vi "Start Battle.vi"(11 "Board Size":i32) -> (0 "Start":bool=TRUE)   [LabVIEW 2015, in "SB SubVIs.lvlib"]
uses:
  SB SubVIs.lvlib
  Type Defs/Square Cluster.ctl
  Square/Square.lvclass
  Globals.vi
  Globals (private).vi
  Type Defs/SB Type Defs.lvlib
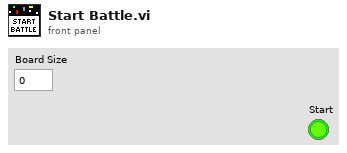
[diagram p1: front panel]
types:
  T1 = typedef "SB Type Defs.lvlib/Square Cluster.ctl" = cluster{"Attacked":bool, "Team":i32, "Next Turn":i32, "DVR":refnum<data-value>}
  T2 = typedef "SB Type Defs.lvlib/UI Refs.ctl" = cluster{"Battlefield":refnum<vi>, "Dashboard":refnum<vi>, "End Battle":refnum<vi>, "Time Limit":refnum<vi>}
  T3 = typedef "SB Type Defs.lvlib/Dashboard.ctl" = cluster{"Color":u32, "Player":i32, "Status":string, "Stats":string}
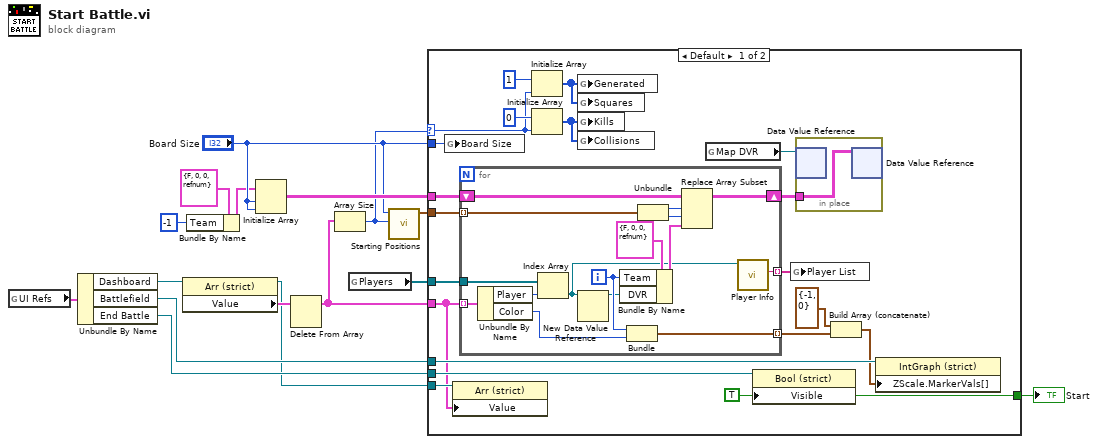
[diagram p0: block diagram]
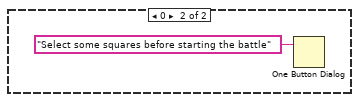
[diagram p2: hidden frame]
diagram:
  n1 = global read "Globals.vi" "UI Refs"() -> (w16:T2)
  n2 = Unbundle By Name(w16) -> ("Dashboard"=w15:refnum<vi>, "Battlefield"=w12:refnum<vi>, "End Battle"=w11:refnum<vi>)
  n3 = property class="Arr (strict)"(reference=w15) -> (reference out=w5:refnum<vi>, "Value"=w10:T3[])  [unwired: 1 in, 1 out]
  n4 = Bundle By Name(cluster=T1 {"Attacked"=FALSE, "Team"=0, "Next Turn"=0, "DVR"=refnum} ("Cluster"), "Team"=-1) -> (w3:T1)
  n5 = Initialize Array(w3, "Board Size", "Board Size") -> (w13:T1[][])
  n6 = Delete From Array(array=w10) -> (array with subset deleted=w6:T3[])  [unwired: 2 in, 1 out]
  n7 = Array Size(array=w6) -> (size(s)=w1:i32)
  n8 = global read "Globals (private).vi" "Players"() -> (w8:refnum<class "Square.lvclass">[])
  n9 = call "Starting Positions.vi"("Player Count"=w1, "Size"="Board Size") -> ("Positions[]"=w14:cluster{i32, i32}[])  [unwired: 9 in]
  n10 = case shown="Default" w1 {
    selector: w1 -> [w21 _]
    tunnel: w14 -> [w36 _]
    tunnel: w13 -> [w35 _]
    tunnel: w12 -> [w34 _]
    tunnel: w11 -> [w30 _]
    tunnel: w6 -> [w23 _]
    tunnel: "Board Size" -> [w27 _]
    tunnel: w8 -> [w26 _]
    tunnel: [w25 _] -> w7
    tunnel: w5 -> [w24 _]
    frame Default {
      w25 = TRUE ("Visible")
      n11 = global write "Globals (private).vi" "Board Size"(w27) -> ()
      n12 = property class="Arr (strict)"(reference=w24, "Value"=w23) -> ()  [unwired: 1 in, 2 out]
      n13 = for {
        tunnel: w36 -> [w50] mode=indexing
        tunnel: w23 -> [w43] mode=indexing
        shift-right: [w51] -> w28
        shift-left: w35 -> [w52]
        tunnel: w26 -> [w45]
        tunnel: [w40] -> w33 mode=indexing
        tunnel: [w37] -> w17 mode=indexing
        i -> [w42]
        n14 = Unbundle By Name(w43) -> ("Player"=w44:i32, "Color"=w41:u32)
        n15 = Index Array(array=w45, index=w44) -> (element=w38:refnum<class "Square.lvclass">)
        n16 = New Data Value Reference(data value=w38) -> (data value reference=w39:refnum<data-value>)  [unwired: 1 in, 1 out]
        n17 = Bundle By Name(cluster=T1 {"Attacked"=FALSE, "Team"=0, "Next Turn"=0, "DVR"=refnum} ("Cluster"), "Team"=w42, "DVR"=w39) -> (w46:T1)
        n18 = Bundle(w42, "Color"=w41) -> (w40:cluster{i32, "Color":u32})  [unwired: 1 in]
        n19 = Unbundle(w50) -> (w49:i32, w48:i32)
        n20 = Replace Array Subset(array=w52, new element=w46, index (row)=w49, index (col)=w48) -> (w51:T1[][])
        n21 = call-dynamic "Player Info.vi"("Square in"=w38) -> ("Name"=w37:string)  [unwired: 7 in, 3 out]
      }
      n22 = Initialize Array(1, w21) -> (w19:i32[])
      n23 = Initialize Array(0, w21) -> (w18:i32[])
      n24 = global write "Globals (private).vi" "Generated"(w19) -> ()
      n25 = global write "Globals (private).vi" "Squares"(w19) -> ()
      n26 = global write "Globals (private).vi" "Kills"(w18) -> ()
      n27 = global write "Globals (private).vi" "Collisions"(w18) -> ()
      n28 = global read "Globals.vi" "Map DVR"() -> (w29:refnum<data-value>)
      n29 = property class="Bool (strict)"(reference=w30, "Visible"=w25) -> ()  [unwired: 1 in, 2 out]
      n30 = global write "Globals (private).vi" "Player List"(w17) -> ()
      n31 = in-place {
        in-place-border: w28 -> [w53]
        n32 = in-place-dvr #1(w29) -> ()  [unwired: 2 out]
        n33 = in-place-dvr #1(w53) -> ()  [unwired: 2 out]
      }
      n34 = Build Array (concatenate)(cluster{i32, u32} {-1, 0} ("output cluster"), w33) -> (w31:cluster{i32, "Color":u32}[])
      n35 = property class="IntGraph (strict)"(reference=w34, "ZScale.MarkerVals[]"=w31) -> ()  [unwired: 1 in, 2 out]
    }
    frame 0 {
      n36 = One Button Dialog(message="Select some squares before starting the battle") -> ()  [unwired: 1 in, 1 out]
    }
  }
  "Start" <- w7
